vi "Write Data to File.vi"(10 "Data":string[](array[string]), 11 "File Path":path) -> ()   [LabVIEW 2013]
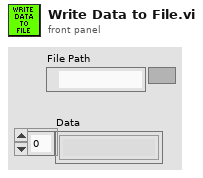
[diagram p1: front panel]
types:
  T1 = enum16{"open", "replace", "create", "open or create", "replace or create", "replace or create with confirmation"}
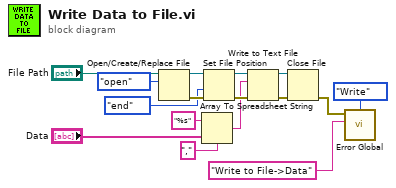
[diagram p0: block diagram]
diagram:
  n1 = Open/Create/Replace File(file path (use dialog)="File Path", operation (0:open)=T1."open") -> (refnum out=w11:refnum<file>, error out=w10:errorcluster)  [unwired: 4 in, 1 out]
  n2 = Array To Spreadsheet String(delimiter (Tab)=",", array="Data", 3:"%s" ("format string")) -> (spreadsheet string=w4:string)
  n3 = Set File Position(refnum=w11, from (0:start)=enum16{"start", "end", "current"}."end", error in=w10) -> (refnum out=w8:refnum<file>, error out=w7:errorcluster)  [unwired: 1 in]
  n4 = Write to Text File(file (use dialog)=w8, text=w4, error in=w7) -> (refnum out=w13:refnum<file>, error out=w14:errorcluster)  [unwired: 1 in, 1 out]
  n5 = Close File(refnum=w13, error in=w14) -> (error out=w2:errorcluster)  [unwired: 1 out]
  n6 = call "Error Global.vi"("Mode"=enum16{"Read", "Write", "Clear Error"}."Write", "Error In"=w2, "Location In"="Write to File->Data" ("delimiter (Tab)")) -> ()  [unwired: 6 in, 2 out]
